vi "Register Element.vi"(8 "error in (no error)":errorcluster, 10 "GUI Element":refnum<class "GUI Element.lvclass">, 11 "PluginGUI in":refnum<class "PluginGUI.lvclass">) -> (0 "error out":errorcluster, 3 "PluginGUI out":refnum<class "PluginGUI.lvclass">)   [LabVIEW 2020, in "VolatusGUI.lvlib" / "PluginGUI.lvclass"]
uses:
  PluginGUI.lvclass
  GUI Element/GUI Element.lvclass
  PluginGUI.lvclass/PluginGUI.ctl
  GUI Element/GUI Element.lvclass/GUI Element.ctl
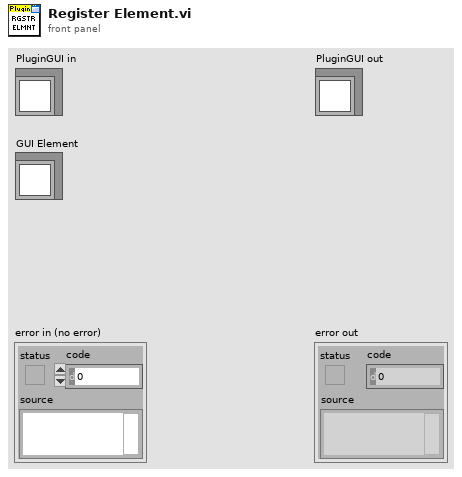
[diagram p1: front panel]
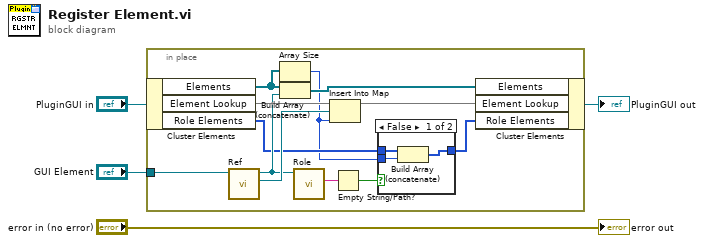
[diagram p0: block diagram]
diagram:
  n1 = in-place {
    in-place-border: "GUI Element" -> [w16]
    n2 = in-place-cluster #1("PluginGUI in") -> ("Elements"=w15:refnum<class "GUI Element.lvclass">[], "Element Lookup"=w14:map{refnum<vi>, i32}, "Role Elements"=w7:i32[])
    n3 = call "Ref.vi"("GUI Element in"=w16) -> ("Ref"=w13:refnum<vi>, "GUI Element out"=w10:refnum<class "GUI Element.lvclass">)  [unwired: 9 in]
    n4 = Array Size(array=w15) -> (size(s)=w6:i32)
    n5 = Build Array (concatenate)(w15, w10) -> (w11:refnum<class "GUI Element.lvclass">[])
    n6 = call "Role.vi"("GUI Element in"=w10) -> ("Role"=w9:string)  [unwired: 9 in, 1 out]
    n7 = Insert Into Map(map in=w14, key=w13, value=w6) -> (map out=w12:map{refnum<vi>, i32})  [unwired: 2 out]
    n8 = Empty String/Path?(string/path=w9) -> (empty?=w8:bool)
    n9 = case shown="False" w8 {
      tunnel: w7 -> [w19 w20]
      tunnel: w6 -> [w18 _]
      tunnel: [w17 w20] -> w5
      frame False {
        n10 = Build Array (concatenate)(w19, w18) -> (w17:i32[])
      }
      frame True {
      }
    }
    n11 = in-place-cluster #1("Elements"=w11, "Element Lookup"=w12, "Role Elements"=w5) -> (→"PluginGUI out":refnum<class "PluginGUI.lvclass">)
  }
  "error out" <- "error in (no error)"
